vi "fgv_points_buff.vi"(6 "closest in":cluster{"x":dbl, "y":dbl} {"x" format="%.2f"; "y" format="%.2f"}, 7 "cmd":T1, 8 "center in":cluster{"x":dbl, "y":dbl} {"x" format="%.2f"; "y" format="%.2f"}, 9 "looktail in":cluster{"x":dbl, "y":dbl} {"x" format="%.2f"; "y" format="%.2f"}, 10 "lookahead in":cluster{"x":dbl, "y":dbl} {"x" format="%.2f"; "y" format="%.2f"}, 11 "lookahead circle in":cluster{"x":dbl, "y":dbl}[](array[cluster]) {"x" format="%.2f"; "y" format="%.2f"}) -> (0 "center out":cluster{"x":dbl, "y":dbl} {"x" format="%.2f"; "y" format="%.2f"}, 1 "looktail out":cluster{"x":dbl, "y":dbl}={"x"=175166.93900924645, "y"=530393.9371218017} {"x" format="%.2f"; "y" format="%.2f"}, 2 "lookahead out":cluster{"x":dbl, "y":dbl}={"x"=175164.2294114242, "y"=530353.9200809624} {"x" format="%.2f"; "y" format="%.2f"}, 3 "lookahead circle out":cluster{"x":dbl, "y":dbl}[](array[cluster])=[{"x"=175166.93900924645, "y"=530355.9296556674}, {"x"=175166.92889717245, "y"=530356.1354916621}, {"x"=175166.8986583353, "y"=530356.3393453436}, {"x"=175166.84858395148, "y"=530356.5392534896}, {"x"=175166.7791562647, "y"=530356.7332908753}, {"x"=175166.69104390158, "y"=530356.9195888147}, {"x"=175166.58509543227, "y"=530357.0963531567}, {"x"=175166.4623311985, "y"=530357.2618815642}, {"x"=175166.32393348694, "y"=530357.4145799079}, {"x"=175166.17123514318, "y"=530357.5529776195}, {"x"=175166.00570673577, "y"=530357.6757418532}, {"x"=175165.82894239377, "y"=530357.7816903226}, {"x"=175165.6426444544, "y"=530357.8698026857}, {"x"=175165.44860706868, "y"=530357.9392303724}, {"x"=175165.24869892266, "y"=530357.9893047563}, {"x"=175165.04484524112, "y"=530358.0195435934}, {"x"=175164.83900924644, "y"=530358.0296556674}, {"x"=175164.63317325176, "y"=530358.0195435934}, {"x"=175164.42931957022, "y"=530357.9893047563}, {"x"=175164.2294114242, "y"=530357.9392303724}, {"x"=175164.03537403847, "y"=530357.8698026857}, {"x"=175163.8490760991, "y"=530357.7816903226}, {"x"=175163.6723117571, "y"=530357.6757418532}, {"x"=175163.5067833497, "y"=530357.5529776195}, {"x"=175163.35408500594, "y"=530357.4145799079}, {"x"=175163.21568729437, "y"=530357.2618815642}, {"x"=175163.0929230606, "y"=530357.0963531567}, {"x"=175162.9869745913, "y"=530356.9195888147}, {"x"=175162.89886222818, "y"=530356.7332908753}, {"x"=175162.8294345414, "y"=530356.5392534896}, {"x"=175162.77936015758, "y"=530356.3393453436}, {"x"=175162.74912132043, "y"=530356.1354916621}, {"x"=175162.73900924643, "y"=530355.9296556674}, {"x"=175162.74912132043, "y"=530355.7238196727}, {"x"=175162.77936015758, "y"=530355.5199659911}, {"x"=175162.8294345414, "y"=530355.3200578452}, {"x"=175162.89886222818, "y"=530355.1260204595}, {"x"=175162.9869745913, "y"=530354.9397225201}, {"x"=175163.0929230606, "y"=530354.7629581781}, {"x"=175163.21568729437, "y"=530354.5974297706}, {"x"=175163.35408500594, "y"=530354.4447314269}, {"x"=175163.5067833497, "y"=530354.3063337153}, {"x"=175163.6723117571, "y"=530354.1835694816}, {"x"=175163.8490760991, "y"=530354.0776210122}, {"x"=175164.03537403847, "y"=530353.9895086491}, {"x"=175164.2294114242, "y"=530353.9200809624}, {"x"=175164.42931957022, "y"=530353.8700065785}, {"x"=175164.63317325176, "y"=530353.8397677414}, {"x"=175164.83900924644, "y"=530353.8296556674}, {"x"=175165.04484524112, "y"=530353.8397677414}, {"x"=175165.24869892266, "y"=530353.8700065785}, {"x"=175165.44860706868, "y"=530353.9200809624}, {"x"=175165.6426444544, "y"=530353.9895086491}, {"x"=175165.82894239377, "y"=530354.0776210122}, {"x"=175166.00570673577, "y"=530354.1835694816}, {"x"=175166.17123514318, "y"=530354.3063337153}, {"x"=175166.32393348694, "y"=530354.4447314269}, {"x"=175166.4623311985, "y"=530354.5974297706}, {"x"=175166.58509543227, "y"=530354.7629581781}, {"x"=175166.69104390158, "y"=530354.9397225201}, {"x"=175166.7791562647, "y"=530355.1260204595}, {"x"=175166.84858395148, "y"=530355.3200578452}, {"x"=175166.8986583353, "y"=530355.5199659911}, {"x"=175166.92889717245, "y"=530355.7238196727}, {"x"=175166.93900924645, "y"=530355.9296556674}] {"x" format="%.2f"; "y" format="%.2f"}, 4 "closest out":cluster{"x":dbl, "y":dbl})   [LabVIEW 2019]
uses:
  Ctrl/points.ctl
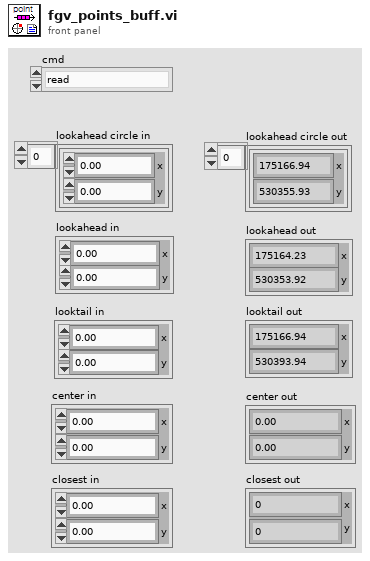
[diagram p1: front panel]
types:
  T1 = typedef "points.ctl" = enum16{"read", "lookahead circle in", "lookahead in", "looktail in", "center in", "closest"}
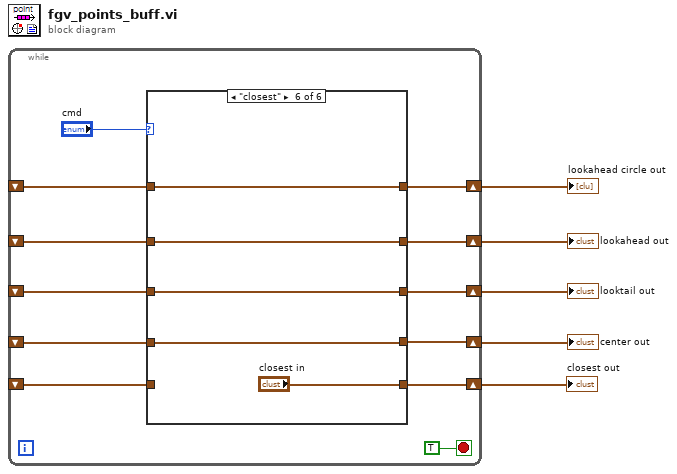
[diagram p0: block diagram]
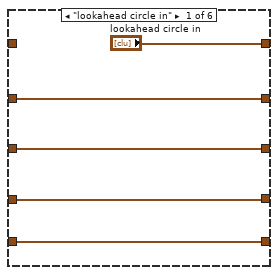
[diagram p2: hidden frame]
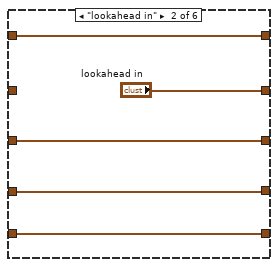
[diagram p3: hidden frame]
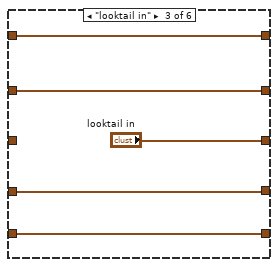
[diagram p4: hidden frame]
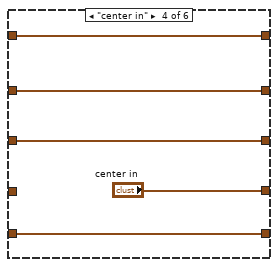
[diagram p5: hidden frame]
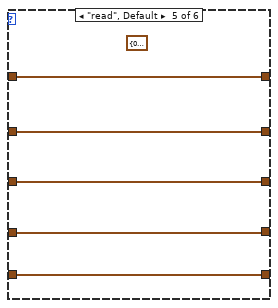
[diagram p6: hidden frame]
diagram:
  n1 = while {
    shift-right: [w15] -> w5
    shift-left: _ -> [w14]
    shift-right: [w13] -> w4
    shift-left: _ -> [w12]
    shift-right: [w11] -> w3
    shift-left: _ -> [w10]
    shift-right: [w9] -> w2
    shift-left: _ -> [w8]
    shift-right: [w7] -> w1
    shift-left: _ -> [w6]
    stop <- TRUE stop-if-true
    n2 = case shown="\"closest\"" "cmd" {
      tunnel: ["lookahead circle in" w27 w32 w37 w42 w44] -> w15
      tunnel: w14 -> [_ w27 w32 w37 w42 w44]
      tunnel: [w21 "lookahead in" w31 w36 w41 w45] -> w13
      tunnel: w12 -> [w21 _ w31 w36 w41 w45]
      tunnel: [w20 w25 "looktail in" w35 w40 w46] -> w11
      tunnel: w10 -> [w20 w25 _ w35 w40 w46]
      tunnel: [w19 w24 w29 "center in" w39 w47] -> w9
      tunnel: w8 -> [w19 w24 w29 _ w39 w47]
      tunnel: [w18 w23 w28 w33 w38 "closest in"] -> w7
      tunnel: w6 -> [w18 w23 w28 w33 w38 _]
      frame "lookahead circle in" {
      }
      frame "lookahead in" {
      }
      frame "looktail in" {
      }
      frame "center in" {
      }
      frame "read", Default {
        (unwired) cluster{"x":dbl, "y":dbl} {"x"=0.0, "y"=0.0} ("true lookahead")
      }
      frame "closest" {
      }
    }
  }
  "lookahead circle out" <- w5
  "lookahead out" <- w4
  "looktail out" <- w3
  "center out" <- w2
  "closest out" <- w1
